vi "getContainer.vi"(8 "error in (no error)":errorcluster, 11 "Theme.Colors in":refnum<class "Theme.Colors.lvclass">) -> (0 "error out":errorcluster, 2 "Container":cluster{"BG":u32, "Hover":u32, "Focused":u32}={"BG"=16119285, "Hover"=15527148, "Focused"=14474460}, 3 "Theme.Colors out":refnum<class "Theme.Colors.lvclass">)   [LabVIEW 2017, in "Theme.lvlib" / "Theme.Colors.lvclass"]
uses:
  Theme.Colors.lvclass
  Theme.Colors.lvclass/Theme.Colors.ctl
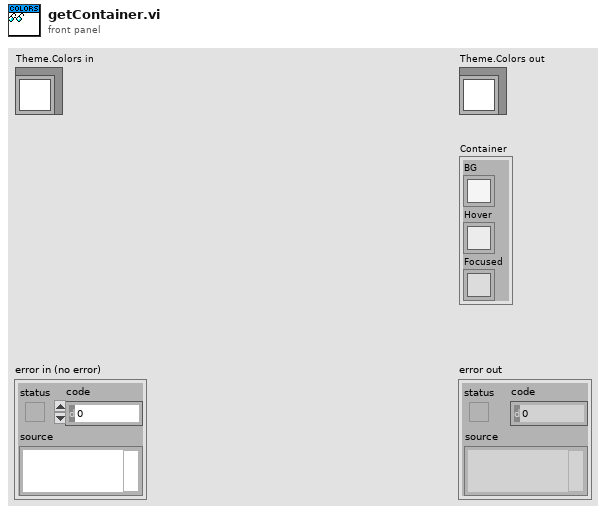
[diagram p1: front panel]
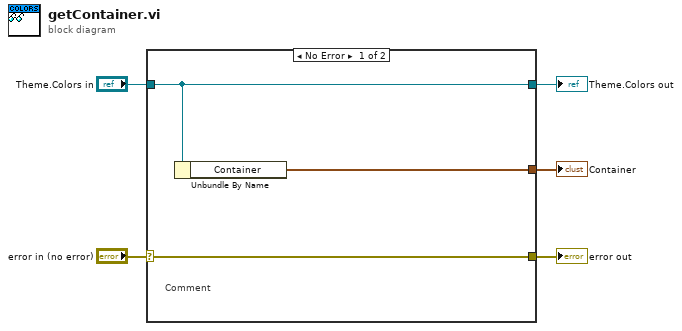
[diagram p0: block diagram]
diagram:
  n1 = case shown="No Error" "error in (no error)" {
    selector: "error in (no error)" -> [w8 w9]
    tunnel: [w8 w9] -> w4
    tunnel: [w7 w10] -> w2
    tunnel: "Theme.Colors in" -> [w7 w10]
    tunnel: [w6 _] -> w1
    frame No Error {
      # "Comment"
      n2 = Unbundle By Name(w7) -> ("Container"=w6:cluster{"BG":u32, "Hover":u32, "Focused":u32})
    }
    frame Error {
    }
  }
  "error out" <- w4
  "Theme.Colors out" <- w2
  "Container" <- w1
